vi "ukol1.vi"() -> ()   [LabVIEW 2022 SP3]
panel:
  in  "stop":bool
  out "Soucet 2":i32
  out "Soucet":dbl
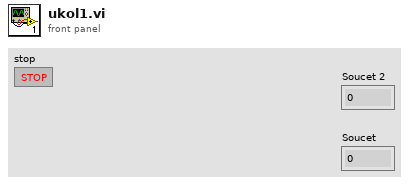
[diagram p1: front panel]
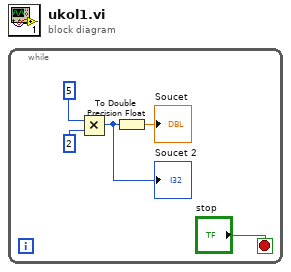
[diagram p0: block diagram]
diagram:
  n1 = while {
    stop <- "stop" stop-if-true
    n2 = Multiply(x=5 ("Cislo 1"), y=2 ("Cislo 2")) -> (x*y=w2:i32)
    "Soucet 2" <- w2
    n3 = To Double Precision Float(number=w2) -> (double precision float=→"Soucet":dbl)
  }
